vi "IPS120 WH4 - Remote Mode.vi"(0 "Remote Mode":bool, 1 "GPIB Address":string) -> ()   [LabVIEW 2009]
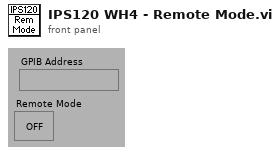
[diagram p1: front panel]
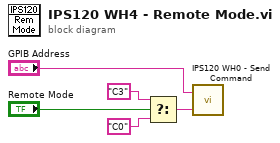
[diagram p0: block diagram]
diagram:
  n1 = Select(t="C3", s="Remote Mode", f="C0") -> (s? t:f=w2:string)
  n2 = call "IPS120 WH0 - Send Command.vi"("Command String"=w2, "GPIB Address"="GPIB Address") -> ()  [unwired: 1 out]
